vi "usbpt104+usbTC-arduino control PWM (concurrent3).vi"(5 "handle":i16, 11 "Units":enum16{"C°", "F°", "K°", "R°"}(ring)) -> (0 "CH 3":sgl, 1 "CH 2":sgl, 2 "CH 0":sgl, 3 "CH 1":sgl, 4 "handle 2":i16, 6 "CH 4":sgl, 7 "CH 8":sgl, 8 "CH 5":sgl, 9 "CH 6":sgl, 10 "CH 7":sgl)   [LabVIEW 2015]
uses:
  usbtc08.dll
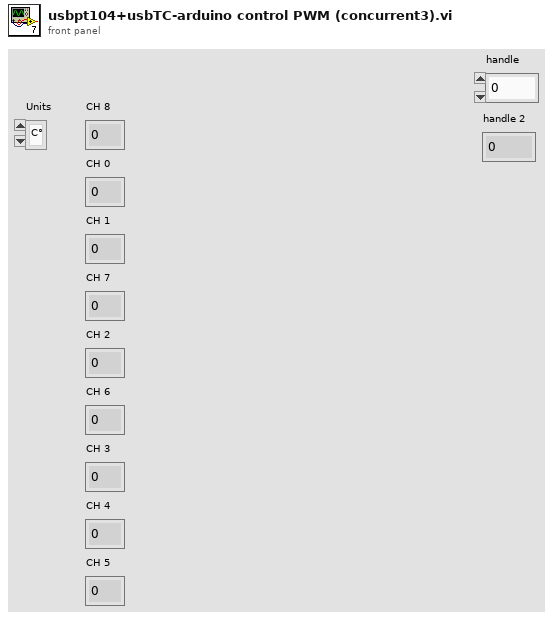
[diagram p1: front panel]
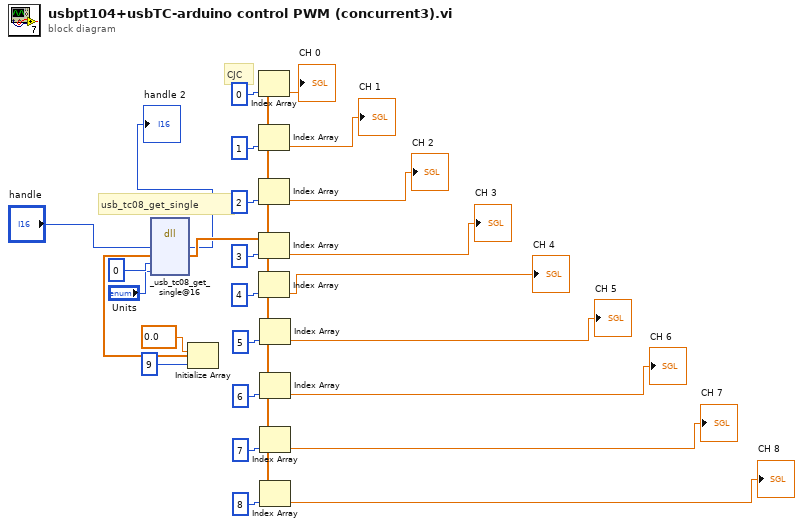
[diagram p0: block diagram]
diagram:
  # "CJC"
  # "usb_tc08_get_single"
  n1 = Initialize Array(sgl 0.0, i16 9) -> (w4:sgl[])
  n2 = dll-call lib="usbtc08.dll" fn="_usb_tc08_get_single@16"("handle"="handle", "temp_buffer"=w4, "overflow"=i16 0, "units"="Units") -> ("handle"=→"handle 2":i16, "temp_buffer"=w3:sgl[])  [unwired: 6 in, 2 out]
  n3 = Index Array(array=w3, index=i16 0) -> (element=→"CH 0":sgl)
  n4 = Index Array(array=w3, index=i16 1) -> (element=→"CH 1":sgl)
  n5 = Index Array(array=w3, index=2) -> (element=→"CH 2":sgl)
  n6 = Index Array(array=w3, index=i16 3) -> (element=→"CH 3":sgl)
  n7 = Index Array(array=w3, index=i16 4) -> (element=→"CH 4":sgl)
  n8 = Index Array(array=w3, index=i16 5) -> (element=→"CH 5":sgl)
  n9 = Index Array(array=w3, index=i16 6) -> (element=→"CH 6":sgl)
  n10 = Index Array(array=w3, index=i16 7) -> (element=→"CH 7":sgl)
  n11 = Index Array(array=w3, index=8) -> (element=→"CH 8":sgl)
